vi "Write Index.vi"(8 "error in (no error)":errorcluster, 10 "Index":i32, 11 "SCD in":refnum<class "SCD.lvclass">) -> (0 "error out":errorcluster, 3 "SCD out":refnum<class "SCD.lvclass">)   [LabVIEW 2023, in "SCD.lvclass"]
doc: "Accessor VI for this class property."
uses:
  SCD.lvclass
  GenericDevice/GenericDevice.lvclass
panel:
  # "Connector Pane"
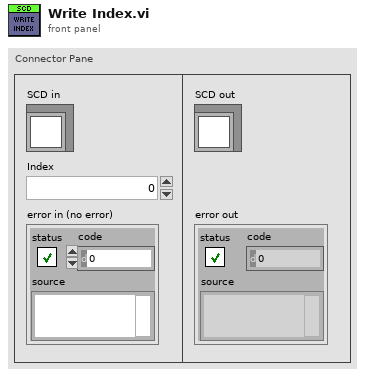
[diagram p1: front panel]
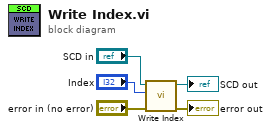
[diagram p0: block diagram]
diagram:
  n1 = call-parent "Write Index.vi"("error in (no error)"="error in (no error)", "Index"="Index", "GenericDevice in"="SCD in") -> ("error out"=→"error out":errorcluster, "GenericDevice out"=→"SCD out":refnum<class "SCD.lvclass">)  [unwired: 7 in]
